vi "mlink_ai_read.vi"(5 "mode":u8[](array[numeric]), 6 "channels":u8[](array[numeric]), 7 "range":dbl[](array[numeric]), 8 "error in (no error)":errorcluster, 11 "connection ID":i32=-1) -> (0 "error out":errorcluster, 2 "data out":dbl[](array[numeric]), 3 "connection ID out":i32)   [LabVIEW 2009, in "MicroDAQ.lvlib" / "mlink.lvlib"]
doc: "This function returns immediately acquired values from MicroDAQ input channels as a 1-by-n array of doubles. The values are stored in an array pointed by data, where n is the number of input channels. The ch_count argument determines number of used channels. The channels \nargument is an array containing channels numbers according to MicroDAQ hardware \nconfiguration. The range argument specifies channel measurement input range. An array n-by-2 where n is number of used channels shall be provided. In order to obtain supported ranges check your ADC configuration. The mode argument specifies measurement mode - differential or single-ended. An mode array of mode settings for used channels shall be provided."
uses:
  <instrlib>/MicroDAQ/Mlink library wraper/mlink.lvlib
  <instrlib>/MicroDAQ/MLink32.dll
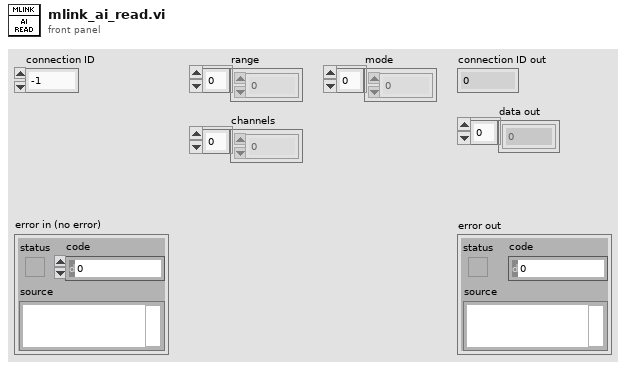
[diagram p1: front panel]
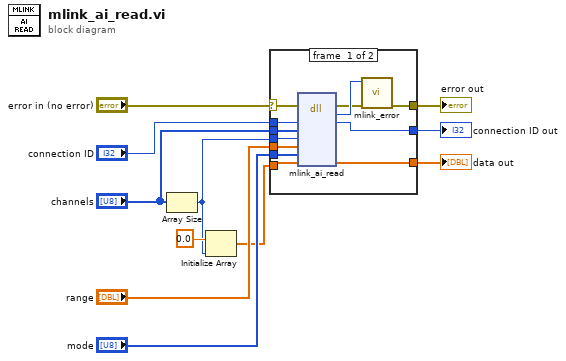
[diagram p0: block diagram]
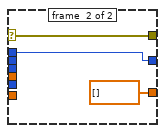
[diagram p2: hidden frame]
diagram:
  n1 = Array Size(array="channels") -> (size(s)=w2:i32)
  n2 = Initialize Array(0.0, w2) -> (w1:dbl[])
  n3 = case shown="No Error" "error in (no error)" {
    selector: "error in (no error)" -> [w21 w26]
    tunnel: "connection ID" -> [w23 w25]
    tunnel: [w22 w25] -> w10
    tunnel: [w18 w26] -> w5
    tunnel: "channels" -> [w17 _]
    tunnel: "range" -> [w16 _]
    tunnel: "mode" -> [w15 _]
    tunnel: [w14 dbl[] [] ("data")] -> w6
    tunnel: w2 -> [w13 _]
    tunnel: w1 -> [w12 _]
    frame #0 {
      n4 = dll-call lib="C:/Program Files (x86)/National Instruments/LabVIEW 2009/instr.lib/MicroDAQ/MLink32.dll" fn="mlink_ai_read"(error in=w21, "connection ID"=w23, "channels"=w17, "count"=w13, "range"=w16, "mode"=w15, "data"=w12) -> (error out=w19:errorcluster, "return type"=w20:i32, "connection ID"=w22:i32, "data"=w14:dbl[])  [unwired: 6 in, 1 out]
      n5 = call <instrlib>:"mlink_error.vi"("error in (no error)"=w19, "error code"=w20) -> ("error out"=w18:errorcluster)  [unwired: 9 in]
    }
    frame #1 {
    }
  }
  "connection ID out" <- w10
  "data out" <- w6
  "error out" <- w5
